vi "Verity_Attenuators.vi"(9 "Switches":i32[](array[numeric]), 10 "nSwitches":i32, 11 "Base Switch ID":i32) -> (3 "Verfied":bool)   [LabVIEW 2012]
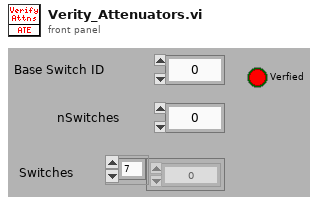
[diagram p1: front panel]
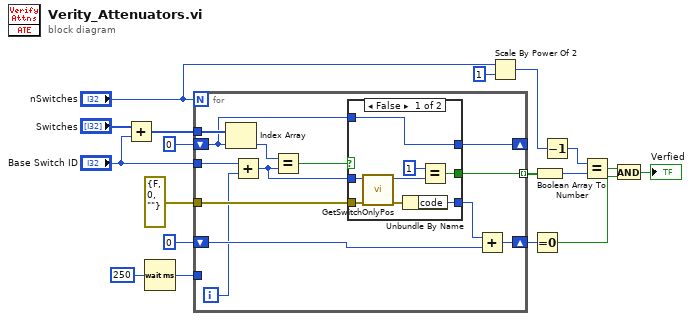
[diagram p0: block diagram]
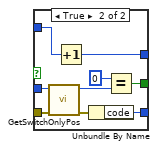
[diagram p2: hidden frame]
diagram:
  n1 = Add(x="Switches", y="Base Switch ID") -> (x+y=w1:i32[])
  n2 = Wait (ms)(milliseconds to wait=u32 250) -> (millisecond timer value=w9:u32)
  n3 = for {
    N: "nSwitches" -> [_]
    tunnel: "Base Switch ID" -> [w31]
    tunnel: errorcluster {"status"=FALSE, "code"=0, "source"=""} ("error in") -> [w30]
    tunnel: [w29] -> w17 mode=indexing
    shift-right: [w25] -> w14
    shift-left: 0 -> [w27]
    tunnel: w9 -> [_]
    tunnel: w1 -> [w23]
    shift-right: [w19] -> _
    shift-left: 0 ("index") -> [w20]
    i -> [w24]
    n4 = Index Array(array=w23, index=w20) -> (element=w22:i32)
    n5 = Add(x=w31, y=w24) -> (x+y=w28:i32)
    n6 = Equal?(x=w22, y=w28) -> (x = y?=w21:bool)
    n7 = case shown="False" w21 {
      tunnel: [w35 w46] -> w29
      tunnel: w28 -> [w37 w45]
      tunnel: w30 -> [w36 w44]
      tunnel: [w33 w42] -> w26
      tunnel: w20 -> [w32 w40]
      tunnel: [w32 w41] -> w19
      frame False {
        n8 = call "GetSwitchOnlyPos.vi"("error in (no error)"=w36, "Circuit ID"=w37) -> ("Error out"=w34:errorcluster, "Position (0=open, 1=closed)"=w38:i32)  [unwired: 4 in]
        n9 = Unbundle By Name(w34) -> ("code"=w33:i32)
        n10 = Equal?(x=1 ("Position (0=open, 1=closed)"), y=w38) -> (x = y?=w35:bool)
      }
      frame True {
        n11 = call "GetSwitchOnlyPos.vi"("error in (no error)"=w44, "Circuit ID"=w45) -> ("Error out"=w43:errorcluster, "Position (0=open, 1=closed)"=w48:i32)  [unwired: 4 in]
        n12 = Increment(x=w40) -> (x+1=w41:i32)
        n13 = Unbundle By Name(w43) -> ("code"=w42:i32)
        n14 = Equal?(x=0 ("Position (0=open, 1=closed)"), y=w48) -> (x = y?=w46:bool)
      }
    }
    n15 = Add(x=w26, y=w27) -> (x+y=w25:i32)
  }
  n16 = Scale By Power Of 2(n="nSwitches", x=u32 1) -> (x*2^n=w5:u32)
  n17 = Equal To 0?(x=w14) -> (x = 0?=w12:bool)
  n18 = Boolean Array To Number(Boolean array=w17) -> (number=w16:u32)
  n19 = Decrement(x=w5) -> (x-1=w4:u32)
  n20 = Equal?(x=w4, y=w16) -> (x = y?=w13:bool)
  n21 = And(x=w13, y=w12) -> (x .and. y?=→"Verfied":bool)
